vi "LVData_initialize.vi"(0 "LVData in":refnum<class "LVData.lvclass">, 1 "FilePath":path, 5 "Activate":bool, 7 "Setting":T1, 11 "error in (no error)":errorcluster) -> (4 "LVData out":refnum<class "LVData.lvclass">, 15 "error out":errorcluster)   [LabVIEW 2020, in "LVData.lvclass"]
uses:
  LVData.lvclass
  ctl/DataSetting.ctl
  LVData.lvclass/LVData.ctl
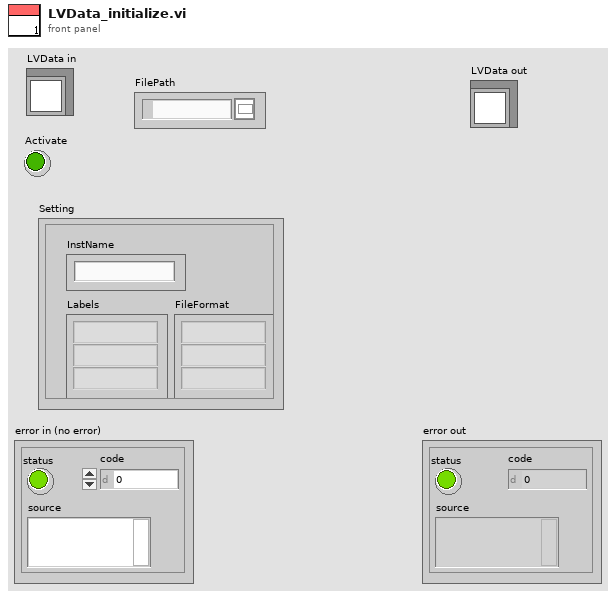
[diagram p1: front panel]
types:
  T1 = typedef "DataSetting.ctl" = cluster{"Labels":string[], "InstName":string, "FileFormat":string[]}
  T2 = enum16{"open", "replace", "create", "open or create", "replace or create", "replace or create with confirmation"}
  T3 = enum16{"Intialized", "Waiting", "Measuring", "Terminated"}
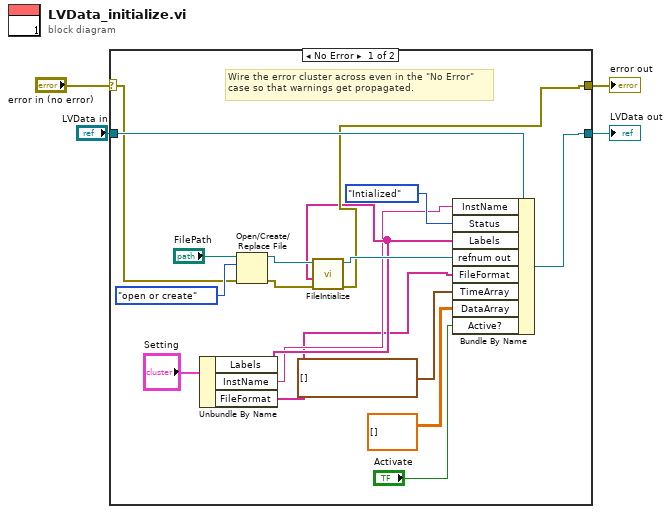
[diagram p0: block diagram]
diagram:
  n1 = case shown="No Error" "error in (no error)" {
    selector: "error in (no error)" -> [w13 w23]
    tunnel: [w9 w23] -> w3
    tunnel: [w14 w22] -> w1
    tunnel: "LVData in" -> [w21 w22]
    frame No Error {
      # "Wire the error cluster across even in the \"No Error\"\ncase so that warnings get propagated."
      n2 = Unbundle By Name("Setting") -> ("Labels"=w7:string[], "InstName"=w6:string, "FileFormat"=w5:string[])
      n3 = Open/Create/Replace File(file path (use dialog)="FilePath", error in=w13, operation (0:open)=T2."open or create") -> (refnum out=w12:refnum<file>, error out=w11:errorcluster)  [unwired: 3 in, 1 out]
      n4 = call "FileIntialize.vi"("Error In"=w11, "Labels"=w7, "refnum in"=w12) -> ("Error Out"=w9:errorcluster, "File Refnum"=w10:refnum<file>)  [unwired: 7 in]
      n5 = Bundle By Name(cluster=w21, "InstName"=w6, "Status"=T3."Intialized", "Labels"=w7, "refnum out"=w10, "FileFormat"=w5, "TimeArray"=timestamp[] [], "DataArray"=dbl[][] [], "Active?"="Activate") -> (w14:refnum<class "LVData.lvclass">)
    }
    frame Error {
    }
  }
  "error out" <- w3
  "LVData out" <- w1
